vi "HFRR ADV v10.vi"() -> ()   [LabVIEW 2025] (continued)
        n1009 = property on="Analysis" class="Bool (strict)"("DisabledEnum"=w969) -> ()  [unwired: 2 in, 2 out]
        n1010 = property on="Home" class="Bool (strict)"("DisabledEnum"=w969) -> ()  [unwired: 2 in, 2 out]
        n1011 = property on="Report" class="Bool (strict)"("DisabledEnum"=w969) -> ()  [unwired: 2 in, 2 out]
        n1012 = property on="Test Setup" class="Bool (strict)"("DisabledEnum"=w969) -> ()  [unwired: 2 in, 2 out]
        n1013 = local read "Service Password enable"() -> (w967:bool)
        n1014 = case shown="True" w967 {
          tunnel: [T16."Disabled" ("Disabled") T16."Enabled" ("Disabled")] -> w966
          frame False {
          }
          frame True {
          }
        }
        n1015 = property on="About" class="Bool (strict)"("DisabledEnum"=w966) -> ()  [unwired: 2 in, 2 out]
      }
      frame "Adv Scar Report" {
        w974 = T16."Enabled" ("Disabled")
        n1016 = property on="Dashboard" class="Bool (strict)"("DisabledEnum"=T16."Disabled" ("Disabled")) -> ()  [unwired: 2 in, 2 out]
        n1017 = property on="Imaging" class="Bool (strict)"("DisabledEnum"=w974) -> ()  [unwired: 2 in, 2 out]
        n1018 = property on="Analysis" class="Bool (strict)"("DisabledEnum"=w974) -> ()  [unwired: 2 in, 2 out]
        n1019 = property on="Home" class="Bool (strict)"("DisabledEnum"=w974) -> ()  [unwired: 2 in, 2 out]
        n1020 = property on="Report" class="Bool (strict)"("DisabledEnum"=w974) -> ()  [unwired: 2 in, 2 out]
        n1021 = property on="Test Setup" class="Bool (strict)"("DisabledEnum"=w974) -> ()  [unwired: 2 in, 2 out]
        n1022 = local read "Service Password enable"() -> (w973:bool)
        n1023 = case shown="True" w973 {
          tunnel: [T16."Disabled" ("Disabled") T16."Enabled" ("Disabled")] -> w972
          frame False {
          }
          frame True {
          }
        }
        n1024 = property on="About" class="Bool (strict)"("DisabledEnum"=w972) -> ()  [unwired: 2 in, 2 out]
      }
      frame "Compare Files" {
        w980 = T16."Enabled" ("Disabled")
        n1025 = local read "Service Password enable"() -> (w979:bool)
        n1026 = property on="Dashboard" class="Bool (strict)"("DisabledEnum"=T16."Disabled" ("Disabled")) -> ()  [unwired: 2 in, 2 out]
        n1027 = property on="Imaging" class="Bool (strict)"("DisabledEnum"=w980) -> ()  [unwired: 2 in, 2 out]
        n1028 = property on="Analysis" class="Bool (strict)"("DisabledEnum"=w980) -> ()  [unwired: 2 in, 2 out]
        n1029 = property on="Home" class="Bool (strict)"("DisabledEnum"=w980) -> ()  [unwired: 2 in, 2 out]
        n1030 = property on="Report" class="Bool (strict)"("DisabledEnum"=w980) -> ()  [unwired: 2 in, 2 out]
        n1031 = property on="Test Setup" class="Bool (strict)"("DisabledEnum"=w980) -> ()  [unwired: 2 in, 2 out]
        n1032 = case shown="True" w979 {
          tunnel: [T16."Disabled" ("Disabled") T16."Enabled" ("Disabled")] -> w978
          frame False {
          }
          frame True {
          }
        }
        n1033 = property on="About" class="Bool (strict)"("DisabledEnum"=w978) -> ()  [unwired: 2 in, 2 out]
      }
      frame "Acquire" {
        n1034 = local read "Service Password enable"() -> (w984:bool)
        n1035 = property on="Test Setup" class="Bool (strict)"("DisabledEnum"=T16."Disabled" ("Disabled")) -> ()  [unwired: 2 in, 2 out]
        n1036 = local read "Auto Start Test"() -> (w986:bool)
        n1037 = local read "RUN"() -> (w988:bool)
        n1038 = case shown="True" w984 {
          tunnel: [T16."Disabled" ("Disabled") T16."Enabled" ("Disabled")] -> w985
          frame False {
          }
          frame True {
          }
        }
        n1039 = Or(x=w988, y=w986) -> (x .or. y?=w987:bool)
        n1040 = case shown="True" w987 {
          tunnel: [T16."Enabled" ("Disabled") T16."Disabled" ("Disabled")] -> w990
          frame False {
          }
          frame True {
          }
        }
        n1041 = property on="About" class="Bool (strict)"("DisabledEnum"=w985) -> ()  [unwired: 2 in, 2 out]
        n1042 = property on="Imaging" class="Bool (strict)"("DisabledEnum"=w990) -> ()  [unwired: 2 in, 2 out]
        n1043 = property on="Dashboard" class="Bool (strict)"("DisabledEnum"=w990) -> ()  [unwired: 2 in, 2 out]
        n1044 = property on="Analysis" class="Bool (strict)"("DisabledEnum"=w990) -> ()  [unwired: 2 in, 2 out]
        n1045 = property on="Home" class="Bool (strict)"("DisabledEnum"=w990) -> ()  [unwired: 2 in, 2 out]
        n1046 = property on="Report" class="Bool (strict)"("DisabledEnum"=w990) -> ()  [unwired: 2 in, 2 out]
      }
      frame "About" {
        n1047 = local read "FILE"() -> (w1003:string)
        n1048 = local read "TEST FILE NAM,E SAVED"() -> (w996:bool)
        n1049 = call <vilib>:"Trim Whitespace.vi"("string"=w1003) -> ("trimmed string"=w1002:string)  [unwired: 1 in]
        n1050 = local read "Auto Start Test"() -> (w1006:bool)
        n1051 = String Length(string=w1002) -> (length=w1001:i32)
        n1052 = Greater?(x=w1001, y=1) -> (0:w998:bool)
        n1053 = And(x=w998, y=w996) -> (x .and. y?=w997:bool)
        n1054 = local read "RUN"() -> (w1008:bool)
        n1055 = case shown="True" w997 {
          tunnel: [T16."Disabled" ("Disabled") T16."Enabled" ("Disabled")] -> w999
          frame False {
          }
          frame True {
          }
        }
        n1056 = Or(x=w1008, y=w1006) -> (x .or. y?=w1007:bool)
        n1057 = property on="About" class="Bool (strict)"("DisabledEnum"=T16."Enabled" ("Disabled")) -> ()  [unwired: 2 in, 2 out]
        n1058 = case shown="False" w1007 {
          tunnel: [T16."Enabled" ("Disabled") T16."Disabled" ("Disabled")] -> w1005
          frame False {
          }
          frame True {
          }
        }
        n1059 = property on="Dashboard" class="Bool (strict)"("DisabledEnum"=w999) -> ()  [unwired: 2 in, 2 out]
        n1060 = property on="Test Setup" class="Bool (strict)"("DisabledEnum"=T16."Disabled" ("Disabled")) -> ()  [unwired: 2 in, 2 out]
        n1061 = property on="Imaging" class="Bool (strict)"("DisabledEnum"=w1005) -> ()  [unwired: 2 in, 2 out]
        n1062 = property on="Analysis" class="Bool (strict)"("DisabledEnum"=w1005) -> ()  [unwired: 2 in, 2 out]
        n1063 = property on="Home" class="Bool (strict)"("DisabledEnum"=w1005) -> ()  [unwired: 2 in, 2 out]
        n1064 = property on="Report" class="Bool (strict)"("DisabledEnum"=w1005) -> ()  [unwired: 2 in, 2 out]
      }
    }
    n1065 = local read "Quit"() -> (w939:bool)
    "Single" <- "Single - Graph"
  }
  n1066 = disable-structure shown="Disabled" {
    disable-tunnel: [w1263 _] -> w36
    disable-tunnel: _ -> [w1262 _]
    frame Disabled {
      n1067 = while {
        tunnel: w1262 -> [_]
        tunnel: [w1264] -> w1263
        tunnel: [w1265] -> _
        i -> [w1265]
        stop <- w1264 stop-if-true
        w1281 = u16 10 items=["1.0"=10, "1.5"=15, "2.0"=20] ("stop bits (10: 1 bit)")
        n1068 = Wait (ms)(milliseconds to wait=u32 10) -> ()  [unwired: 1 out]
        n1069 = call-poly "VISA Configure Serial Port"("VISA resource name"=refnum<visa-resource-name> "ASRL1::INSTR" ("COM PORT"), "timeout (10sec)"=u32 10, "baud rate (9600)"=u32 57600, "data bits (8)"=u16 8, "stop bits (10: 1 bit)"=w1281) -> ("VISA resource name out"=w1267:refnum<visa-resource-name>, "error out"=w1276:errorcluster)  [unwired: 9 in]
        n1070 = VISA Read(VISA resource name=w1267, byte count=u32 2 ("byte count (0)")) -> (read buffer=w1275:string)  [unwired: 1 in, 3 out]
        n1071 = String Subset(string=w1275, offset (0)=0, length (rest)=2 ("length (rest)")) -> (substring=w1274:string)
        n1072 = Match Pattern(string=w1274, regular expression="<>") -> (offset past match=w1271:i32)  [unwired: 1 in, 3 out]
        n1073 = Greater Or Equal?(x=w1271, y=0) -> (x >= y?=w1266:bool)
        n1074 = case shown="True" w1266 {
          tunnel: w1267 -> [_ w1285]
          tunnel: w1276 -> [_ w1284]
          frame False {
          }
          frame True {
            n1075 = VISA Read(VISA resource name=w1285, byte count=u32 32 ("byte count (0)"), error in (no error)=w1284) -> (read buffer=w1283:string)  [unwired: 3 out]
            n1076 = String Subset(string=w1283, offset (0)=0, length (rest)=8 ("length (rest)")) -> (substring=w1287:string)
            n1077 = String Subset(string=w1283, offset (0)=8, length (rest)=8 ("length (rest)")) -> (substring=w1288:string)
            n1078 = Decimal String To Number(string=w1288) -> (number=w1295:i32)  [unwired: 2 in, 1 out]
            n1079 = Decimal String To Number(string=w1287) -> (number=w1291:i32)  [unwired: 2 in, 1 out]
            n1080 = Divide(x=w1295, y=10000) -> ()  [unwired: 1 out]
            n1081 = Divide(x=w1291, y=1000000) -> ()  [unwired: 1 out]
          }
        }
        n1082 = local read "Quit"() -> (w1264:bool)
      }
    }
    frame Enabled {
    }
  }
  n1083 = local write "Err Count"(0 ("Err Count")) -> ()
  n1084 = local write "FRICVALZ"(0.0 ("FRICVALZ")) -> ()
  n1085 = Tick Count (ms)() -> (millisecond timer value=w49:u32)
  n1086 = while {
    shift-right: [w1314] -> w53
    shift-left: _ -> [w1303]
    shift-right: [w1313] -> w52
    shift-left: errorcluster {"status"=TRUE, "code"=0, "source"="Init"} ("error IO") -> [w1305]
    shift-right: [w1311] -> _
    shift-left: w49 -> [w1312]
    tunnel: [w1298] -> w40
    tunnel: [w1310] -> _
    i -> [w1310]
    stop <- w1298 stop-if-true
    n1087 = local read "Com Port 1"() -> (w1304:refnum<visa-resource-name>)
    n1088 = local read "Port 1a"() -> (w1306:bool)
    n1089 = local read "Port 3"() -> (w1307:bool)
    n1090 = Not Equal?(x=w1304, y=w1303) -> (x != y?=w1302:bool)
    n1091 = Or(x=w1307, y=w1306) -> (x .or. y?=w1309:bool)
    n1092 = Unbundle(w1305) -> ("status"=→"Port 3":bool)  [unwired: 2 out]
    n1093 = flat-sequence {
      tunnel: [w1317] -> w1301
      tunnel: w1305 -> [w1317]
      frame #0 {
        n1094 = Wait (ms)(milliseconds to wait=u32 200) -> ()  [unwired: 1 out]
      }
    }
    n1095 = case shown="True" w1309 {
      frame False {
        w1319 = FALSE ("Visible")
        n1096 = property on="Port 1a" class="Bool (strict)"("Visible"=w1319) -> ()  [unwired: 2 in, 2 out]
        n1097 = property on="Port 3" class="Bool (strict)"("Visible"=w1319) -> ()  [unwired: 2 in, 2 out]
      }
      frame True {
        w1320 = TRUE ("Visible")
        n1098 = property on="Port 1a" class="Bool (strict)"("Visible"=w1320) -> ()  [unwired: 2 in, 2 out]
        n1099 = property on="Port 3" class="Bool (strict)"("Visible"=w1320) -> ()  [unwired: 2 in, 2 out]
      }
    }
    n1100 = Or(x=w1302, y="Re-initialize Port1") -> (x .or. y?=w1299:bool)
    n1101 = case shown="True" w1299 {
      tunnel: [w1315 errorcluster {"status"=TRUE, "code"=0, "source"="Init"} ("error out")] -> w1300
      tunnel: w1301 -> [w1315 _]
      frame False {
      }
      frame True {
      }
    }
    n1102 = case shown="No Error" w1300 {
      selector: w1300 -> [w1321 w1666]
      tunnel: [w1326 w1671] -> w1314
      tunnel: [w1325 w1663] -> w1313
      tunnel: w1303 -> [w1324 w1669]
      tunnel: w1312 -> [w1323 w1668]
      tunnel: [w1322 w1668] -> w1311
      frame No Error {
        n1103 = stacked-sequence {
          tunnel: [w1336 _ _ _ _ _] -> w1326
          tunnel: [w1335 _ _ _ _ _] -> w1325
          tunnel: w1324 -> [w1331 _ _ _ _ _]
          tunnel: w1321 -> [w1330 _ _ _ _ _]
          tunnel: w1323 -> [_ w1459 _ _ _ _]
          tunnel: [_ w1458 _ _ _ _] -> w1322
          tunnel: [_ w1430 _ _ _ _] -> _
          frame #0 {
            n1104 = property class="Instr"(reference=w1331, error in=w1330) -> (reference out=w1333:refnum<visa-resource-name>, error out=w1334:errorcluster, "Serial Settings:Number of Bytes at Serial Port"=w1327:u32)
            "Sps 3" <- w1327
            "Port 1" <- w1327
            n1105 = Greater?(x=w1327, y=u32 5) -> (0:w1329:bool)
            n1106 = case shown="True" w1329 {
              tunnel: w1333 -> [w1338 w1365]
              tunnel: w1334 -> [w1337 w1344]
              tunnel: [w1337 w1340] -> w1335
              tunnel: [w1338 w1366] -> w1336
              frame False {
              }
              frame True {
                w1339 = TRUE ("PAUSE")
                w1342 = TRUE ("PAUSE")
                # "Out as Volts"
                n1107 = call "ELAPSED TIMER VI - uno.vi"("error in"=w1344, "RESET"=w1342, "PAUSE"=w1342) -> ("error out"=w1343:errorcluster)  [unwired: 6 in, 2 out]
                n1108 = local read "Residual Uno"() -> (w1359:string)
                n1109 = while {
                  tunnel: [w1414] -> w1341
                  tunnel: [w1413] -> w1366
                  tunnel: w1343 -> [w1412]
                  tunnel: w1365 -> [w1411]
                  tunnel: [w1408] -> _
                  shift-right: [w1404] -> w1347
                  shift-left: w1359 -> [w1406]
                  i -> [w1408]
                  stop <- w1403 stop-if-true
                  w1401 = FALSE ("PAUSE")
                  n1110 = property class="Instr"(reference=w1411, error in=w1412) -> (reference out=w1416:refnum<visa-resource-name>, error out=w1415:errorcluster, "Serial Settings:Number of Bytes at Serial Port"=w1407:u32)
                  n1111 = local read "Quit"() -> (w1402:bool)
                  n1112 = call "ELAPSED TIMER VI - uno.vi"("TARGET"=5.0, "RESET"=w1401, "PAUSE"=w1401) -> ("ELAPSED INDICATION"=w1399:bool)  [unwired: 6 in, 2 out]
                  "ELAPSED INDICATION" <- w1399
                  n1113 = VISA Read(VISA resource name=w1416, byte count=w1407, error in (no error)=w1415) -> (VISA resource name out=w1413:refnum<visa-resource-name>, read buffer=w1405:string, error out=w1414:errorcluster)  [unwired: 1 out]
                  n1114 = Greater?(x=w1407, y=u32 30) -> (0:w1409:bool)
                  n1115 = Concatenate Strings(w1406, w1405) -> (w1404:string)
                  n1116 = Compound Arithmetic op=OR(w1409, w1402, w1399) -> (w1403:bool)
                }
                "UnoRead" <- w1347
                n1117 = call "ELAPSED TIMER VI - uno.vi"("error in"=w1341, "RESET"=w1339, "PAUSE"=w1339) -> ("error out"=w1340:errorcluster)  [unwired: 6 in, 2 out]
                n1118 = while {
                  shift-right: [w1385] -> w1358
                  shift-left: w1347 -> [w1391]
                  tunnel: [w1384] -> w1354 mode=indexing
                  tunnel: [w1386] -> _
                  i -> [w1386]
                  stop <- w1383 stop-if-true
                  n1119 = Match Pattern(string=w1391, regular expression="*") -> (after substring=w1389:string)  [unwired: 1 in, 3 out]
                  n1120 = local read "Quit"() -> (w1382:bool)
                  n1121 = local read "ELAPSED INDICATION"() -> (w1381:bool)
                  n1122 = Match Pattern(string=w1389, regular expression="&") -> (before substring=w1384:string, after substring=w1385:string, offset past match=w1387:i32)  [unwired: 1 in, 1 out]
                  n1123 = Less Than 0?(x=w1387) -> (x < 0?=w1388:bool)
                  n1124 = Compound Arithmetic op=OR(w1388, w1382, w1381) -> (w1383:bool)
                }
                n1125 = local write "Residual Uno"(w1358) -> ()
                n1126 = Array Size(array=w1354) -> (size(s)=w1355:i32)
                n1127 = Decrement(x=w1355) -> (x-1=w1357:i32)
                n1128 = Delete From Array(array=w1354, length=1, index=w1357) -> (array with subset deleted=w1352:string[])  [unwired: 1 out]
                n1129 = Array Size(array=w1352) -> (size(s)=w1351:i32)
                n1130 = Decrement(x=w1351) -> (x-1=w1350:i32)
                n1131 = while {
                  tunnel: [w1380] -> w1363 mode=indexing
                  tunnel: [w1379] -> w1362 mode=indexing
                  tunnel: w1352 -> [w1373] mode=indexing
                  tunnel: w1350 -> [w1372]
                  tunnel: [w1371] -> _
                  i -> [w1371]
                  stop <- w1367 stop-if-true
                  w1374 = 0 ("length (rest)")
                  w1376 = ";" ("regular expression")
                  n1132 = local read "ELAPSED INDICATION"() -> (w1370:bool)
                  n1133 = Less Or Equal?(x=w1372, y=w1371) -> (x <= y?=w1368:bool)
                  n1134 = local read "Quit"() -> (w1369:bool)
                  n1135 = Compound Arithmetic op=OR(w1368, w1369, w1370) -> (w1367:bool)
                  n1136 = Match Pattern(string=w1373, regular expression=w1376) -> (before substring=w1378:string, after substring=w1377:string)  [unwired: 1 in, 2 out]
                  n1137 = Decimal String To Number(string=w1378, default (0L)=w1374) -> (number=w1380:i32)  [unwired: 1 in, 1 out]
                  n1138 = Match Pattern(string=w1377, regular expression=w1376) -> (before substring=w1375:string)  [unwired: 1 in, 3 out]
                  n1139 = Decimal String To Number(string=w1375, default (0L)=w1374) -> (number=w1379:i32)  [unwired: 1 in, 1 out]
                }
                n1140 = case shown="0, Default" "ADC Res" {
                  tunnel: [w1394 w1396] -> w1346
                  frame 0, Default {
                    n1141 = Divide(x=65535 ("length (rest)"), y=2 ("length (rest)")) -> (x/y=w1394:dbl)
                  }
                  frame 1 {
                    n1142 = Divide(x=16777216 ("length (rest)"), y=2 ("length (rest)")) -> (x/y=w1396:dbl)
                  }
                }
                n1143 = Bundle(w1363, w1362) -> (w1353:cluster{i32[], i32[]})  [unwired: 1 in]
                n1144 = Divide(x=w1353, y=w1346) -> (x/y=w1364:cluster{dbl[], dbl[]})
                n1145 = Multiply(x=w1364, y=sgl 5.03 ("Numeric")) -> (x*y=w1361:cluster{dbl[], dbl[]})
                n1146 = Unbundle(w1361) -> (→"Ch1":dbl[], →"Ch0":dbl[])
              }
            }
            n1147 = Not(x=w1329) -> (.not. x?=→"Port 1a":bool)
          }
          frame #1 {
            n1148 = local read "zOff 2"() -> (w1451:dbl)
            n1149 = local read "Ch1"() -> (w1441:dbl[])
            n1150 = case shown="True" "Zero 2" {
              tunnel: w1441 -> [_ w1471]
              frame False {
              }
              frame True {
                n1151 = call-poly <vilib>:"Mean.vi"("X"=w1471) -> ("mean"=→"zOff 2":dbl)  [unwired: 1 out]
                n1152 = local write "Zero 2"(FALSE ("Zero")) -> ()
              }
            }
            n1153 = Subtract(x=w1441, y=w1451) -> (x-y=w1447:dbl[])
            n1154 = call-poly <vilib>:"Mean.vi"("X"=w1441) -> ("mean"=w1442:dbl)  [unwired: 1 out]
            "Slide 3" <- w1442
            n1155 = Multiply(x=w1447, y=1.0 ("PG Oth")) -> (x*y=w1433:dbl[])
            n1156 = local read "FF buffer"() -> (w1438:dbl[])
            n1157 = Divide(x=w1433, y=1) -> (x/y=w1432:dbl[])
            "Fric Val" <- w1432
            n1158 = call <vilib>:"Mean PtByPt.vi"("x"=w1442, "sample length"=10, "initialize"="Reset 2") -> ("mean"=→"Mean Pos Fil 2":dbl)  [unwired: 1 in, 1 out]
            n1159 = Array Size(array=w1438) -> (size(s)=w1440:i32)
            n1160 = call-poly <vilib>:"Mean.vi"("X"=w1432) -> ("mean"=w1446:dbl)  [unwired: 1 out]
            n1161 = Insert Into Array(array=w1438, index=w1440, new element=w1432) -> (w1435:dbl[])
            n1162 = Array Size(array=w1435) -> (size(s)=w1434:i32)
            n1163 = case shown="True" "DC corr 2" {
              tunnel: w1432 -> [w1474 w1477]
              tunnel: [w1474 w1476] -> w1439
              tunnel: w1446 -> [_ w1475]
              frame False {
              }
              frame True {
                n1164 = Subtract(x=w1477, y=w1475) -> (x-y=w1476:dbl[])
              }
            }
            n1165 = Tick Count (ms)() -> (millisecond timer value=w1458:u32)
            n1166 = Greater?(x=w1434, y=1000) -> (0:w1436:bool)
            n1167 = Subtract(x=w1458, y=w1459) -> (x-y=w1457:u32)
            n1168 = case shown="True" w1436 {
              tunnel: [w1464 w1467] -> w1423
              tunnel: w1435 -> [w1464 w1470]
              tunnel: w1434 -> [_ w1469]
              frame False {
              }
              frame True {
                n1169 = Subtract(x=w1469, y=1000) -> (x-y=w1465:i32)
                n1170 = Delete From Array(array=w1470, length=w1465, index=0) -> (array with subset deleted=w1467:dbl[])  [unwired: 1 out]
              }
            }
            n1171 = Divide(x=w1457, y=u32 1000 ("x")) -> (x/y=w1455:dbl)
            n1172 = Array Size(array=w1439) -> (size(s)=w1454:i32)
            n1173 = Divide(x=w1454, y=w1455) -> (x/y=w1450:dbl)
            "Sps 2" <- w1450
            n1174 = Reciprocal(x=w1450) -> (1/x=w1448:dbl)
            "dt" <- w1448
            n1175 = local read "FRIC. FORCE :"() -> (w1420:dbl)
            n1176 = local write "FF buffer"(w1423) -> ()
            n1177 = Negate(x=w1423) -> (-x=w1422:dbl[])
            n1178 = call "Elapsed Time5"("Time Target (s)"="check time s", "Reset"="Reset 3") -> ("Time has Elapsed"=w1425:bool)  [unwired: 10 in, 7 out]
            n1179 = Array Max & Min(array=w1422) -> (max value=w1430:dbl)  [unwired: 3 out]
            n1180 = Bundle By Name("Y"=w1439, "dt"=w1448, "t0"=timestamp(0 s since 1904-01-01)) -> (w1418:waveform(dbl))  [unwired: 1 in]
            n1181 = Multiply(x=w1420, y=21.1986) -> (x*y=w1419:dbl)
            n1182 = Greater Or Equal?(x=w1430, y="Threshold value") -> (x >= y?=w1426:bool)
            n1183 = Multiply(x=w1419, y=w1418) -> (x*y=→"FF_Wfm":waveform(dbl))
            n1184 = And(x=w1426, y=w1425) -> (x .and. y?=w1424:bool)
            n1185 = case shown="True" w1424 {
              frame False {
                n1186 = local write "Reset 3"(FALSE ("Reset 3")) -> ()
              }
              frame True {
                n1187 = local write "Reset 3"(TRUE ("Reset 3")) -> ()
                n1188 = local write "save dpt"(TRUE ("save dpt")) -> ()
              }
            }
          }
          frame #2 {
            n1189 = local read "FF buffer"() -> (w1484:dbl[])
            n1190 = Array Max & Min(array=w1484) -> (max value=w1479:dbl, min value=w1480:dbl)  [unwired: 2 out]
            n1191 = Subtract(x=w1479, y=w1480) -> (x-y=w1481:dbl)
            n1192 = Multiply(x=1.0 ("y 2"), y="Threshold") -> ()  [unwired: 1 out]
            n1193 = Greater?(x=w1481, y="Threshold") -> (0:w1478:bool)
            n1194 = case shown="True" w1478 {
              tunnel: w1484 -> [_ w1491]
              tunnel: [_ w1489] -> _
              frame False {
              }
              frame True {
                w1490 = 1.0 ("y")
                n1195 = Delete From Array(array=w1491, length=100, index=0) -> (deleted portion=w1496:dbl[])  [unwired: 1 out]
                n1196 = call-poly <vilib>:"Mean.vi"("X"=w1496) -> ("mean"=w1495:dbl)  [unwired: 1 out]
                n1197 = Subtract(x=w1491, y=w1495) -> (x-y=w1494:dbl[])
                n1198 = Multiply(x=w1490, y=w1490) -> (x*y=w1492:dbl)
                n1199 = Multiply(x=w1494, y=w1492) -> (x*y=w1493:dbl[])
                "FF cal val" <- w1493
                n1200 = Array Size(array=w1493) -> (size(s)=w1487:i32)
                n1201 = Array Max & Min(array=w1493) -> (max value=w1486:dbl, min value=w1485:dbl)  [unwired: 2 out]
                n1202 = property on="FF Calibration g" class="WFGraph (strict)"("X Scale.Range:Minimum"=0.0 ("y"), "X Scale.Range:Maximum"=w1487, "Y Scale.Range:Minimum"=w1486, "Y Scale.Range:Maximum"=w1485) -> ()  [unwired: 2 in, 2 out]
                n1203 = local read "FRIC. FORCE :"() -> (w1489:dbl)
              }
            }
          }
          frame #3 {
            # "5"
            n1204 = local read "DISPLACEMENT :"() -> (w1587:dbl)
            n1205 = Multiply(x=w1587, y=1.0) -> (x*y=w1505:dbl)
            n1206 = local read "zOff 3"() -> (w1590:dbl)
            n1207 = local read "Ch0"() -> (w1518:dbl[])
            n1208 = case shown="True" "Zero 3" {
              tunnel: w1518 -> [_ w1605]
              frame False {
              }
              frame True {
                n1209 = call-poly <vilib>:"Mean.vi"("X"=w1605) -> ("mean"=→"zOff 3":dbl)  [unwired: 1 out]
                n1210 = local write "Zero 3"(FALSE ("Zero")) -> ()
              }
            }
            n1211 = Add(x=w1518, y="Offset") -> (x+y=w1517:dbl[])
            n1212 = Multiply(x=w1505, y="DISPLACEMENT : 2") -> (x*y=w1572:dbl)
            n1213 = Subtract(x=w1518, y=w1590) -> (x-y=w1575:dbl[])
            n1214 = Multiply(x=w1575, y=w1572) -> (x*y=w1574:dbl[])
            n1215 = Multiply(x=w1575, y=w1505) -> (x*y=w1586:dbl[])
            "ABS DP" <- w1586
            n1216 = local read "Standard Slip Gauge (mm)"() -> (w1573:dbl)
            n1217 = call-poly <vilib>:"Mean.vi"("X"=w1574) -> ("mean"=w1504:dbl)  [unwired: 1 out]
            "Disp (mm)" <- w1504
            "software msrnt" <- w1504
            n1218 = Multiply(x=w1517, y="Gain") -> (x*y=w1512:dbl[])
            "Voltage LVDT Acq" <- w1512
            "gLVDTraw" <- w1512
            n1219 = call-poly <vilib>:"Mean.vi"("X"=w1586) -> ("mean"=w1577:dbl)  [unwired: 1 out]
            n1220 = case shown="True" "DC correction" {
              tunnel: w1586 -> [w1608 w1611]
              tunnel: [w1608 w1610] -> w1524
              tunnel: w1577 -> [_ w1609]
              frame False {
              }
              frame True {
                n1221 = Subtract(x=w1611, y=w1609) -> (x-y=w1610:dbl[])
              }
            }
            n1222 = Divide(x=w1504, y=w1573) -> (x/y=w1571:dbl)
            n1223 = call-poly <vilib>:"Mean.vi"("X"=w1512) -> ("mean"=w1511:dbl)  [unwired: 1 out]
            n1224 = Array Max & Min(array=w1512) -> (max value=w1516:dbl, min value=w1515:dbl)  [unwired: 2 out]
            n1225 = Multiply(x=w1571, y=w1572) -> (x*y=→"DISPLACEMENT : 3":dbl)
            n1226 = Subtract(x=w1516, y=w1515) -> (x-y=→"Pk-Pk":dbl)
            n1227 = local read "dt"() -> (w1589:dbl)
            n1228 = Threshold 1D Array(2:0.0 ("threshold y"), 3:w1524) -> (0:w1541:dbl)  [unwired: 1 in]
            n1229 = Bundle By Name("Y"=w1524, "dt"=w1589, "t0"=timestamp(0 s since 1904-01-01)) -> (w1579:waveform(dbl))  [unwired: 1 in]
            n1230 = local read "FF_Wfm"() -> (w1578:waveform(dbl))
            n1231 = Equal To 0?(x=w1541) -> (x = 0?=w1542:bool)
            n1232 = case shown="True" w1542 {
              tunnel: w1524 -> [_ w1599]
              tunnel: [w1595 w1596] -> w1537
              tunnel: w1541 -> [w1595 _]
              frame False {
              }
              frame True {
                n1233 = Threshold 1D Array(1:20 ("start index (0)"), 2:0.0 ("threshold y"), 3:w1599) -> (0:w1596:dbl)
              }
            }
            n1234 = Build Array(w1579, w1578) -> (w1560:waveform(dbl)[])
            "Waveform Graph 2" <- w1560
            n1235 = call-poly <vilib>:"Extract Single Tone Information.vi"("time signal in"=w1579) -> ("detected amplitude"=w1513:dbl, "detected frequency"=→"RawFreq":dbl)  [unwired: 5 in, 4 out]
            n1236 = Multiply(x=w1513, y=2.0) -> (x*y=w1500:dbl)
            n1237 = Subtract(x=w1511, y="LvdtOff") -> (x-y=w1510:dbl)
            n1238 = local read "StrokeL"() -> (w1501:dbl)
            n1239 = Not A Number/Path/Refnum?(number/path/refnum=w1500) -> (NaN/Path/Refnum?=w1502:bool)
            n1240 = Subtract(x=w1510, y=w1513) -> (x-y=w1522:dbl)
            n1241 = Add(x=w1513, y=w1510) -> (x+y=w1521:dbl)
            n1242 = Index Array(array=w1560) -> (element #1=w1561:waveform(dbl), element #2=w1563:waveform(dbl))  [unwired: 2 in]
            n1243 = Select(t=w1501, s=w1502, f=w1500) -> (s? t:f=w1499:dbl)
            "Stroke" <- w1499
            "Mean(RAW) Stroke" <- w1499
            "StrokeL" <- w1499
            n1244 = Bundle(w1510, w1522, w1521) -> (→"Slide 8":cluster{dbl, dbl, dbl})  [unwired: 1 in]
            n1245 = Unbundle By Name(w1561) -> ("Y"=w1534:dbl[])
            n1246 = Split 1D Array(array=w1524, index=w1537) -> (second subarray=w1538:dbl[])  [unwired: 1 out]
            n1247 = In Range and Coerce(upper limit=1.5, x=w1499, lower limit=0.5) -> (In Range?=w1583:bool)  [unwired: 1 out]
            n1248 = Split 1D Array(array=w1534, index="Window") -> (second subarray=w1552:dbl[])  [unwired: 1 out]
            n1249 = Unbundle By Name(w1563) -> ("Y"=w1535:dbl[])
            n1250 = Threshold 1D Array(1:180 ("start index (0)"), 2:0.0 ("threshold y"), 3:w1538) -> (0:w1536:dbl)
            n1251 = local read "Test \nStatus"() -> (w1580:bool)
            n1252 = Split 1D Array(array=w1535, index=w1537) -> (second subarray=w1532:dbl[])  [unwired: 1 out]
            n1253 = Not(x=w1583) -> (.not. x?=w1582:bool)
            n1254 = call-poly <vilib>:"RMS.vi"("X"=w1552) -> ("rms value"=w1508:dbl)  [unwired: 1 out]
            "Current (A)" <- w1508
            n1255 = Array Max & Min(array=w1552) -> (max value=w1566:dbl, min value=w1567:dbl)  [unwired: 2 out]
            n1256 = Array Max & Min(array=w1535) -> (max value=w1564:dbl, min value=w1565:dbl)  [unwired: 2 out]
            n1257 = Subtract(x=w1566, y=w1567) -> (x-y=w1568:dbl)
            n1258 = Subtract(x=w1564, y=w1565) -> (x-y=w1569:dbl)
            n1259 = And(x=w1582, y=w1580) -> (x .and. y?=w1581:bool)
            n1260 = Split 1D Array(array=w1538, index=w1536) -> (first subarray=w1531:dbl[])  [unwired: 1 out]
            n1261 = Split 1D Array(array=w1532, index=w1536) -> (first subarray=w1529:dbl[])  [unwired: 1 out]
            n1262 = case shown="True" w1581 {
              tunnel: [i32[] [] w1601] -> _
              frame False {
              }
              frame True {
                n1263 = local read "UnoRead"() -> (w1603:string)
                n1264 = local read "Array"() -> (w1604:string[])
                n1265 = Build Array (concatenate)(w1604, w1603) -> (w1602:string[])
                "Array" <- w1602
                n1266 = String Length(string=w1602) -> (length=w1601:i32[])
              }
            }
            n1267 = local read "G_val"() -> (w1554:dbl)
            n1268 = Divide(x=w1569, y=w1568) -> (x/y=w1557:dbl)
            n1269 = call-poly <vilib>:"RMS.vi"("X"=w1529) -> ("rms value"=w1553:dbl)  [unwired: 1 out]
            n1270 = call-poly <vilib>:"Hanning Window.vi"("X"=w1531) -> ("Windowed X"=w1530:dbl[])  [unwired: 1 out]
            n1271 = call-poly <vilib>:"Hanning Window.vi"("X"=w1529) -> ("Windowed X"=w1528:dbl[])  [unwired: 1 out]
            n1272 = local read "Constant (G)"() -> (w1546:dbl)
            n1273 = Divide(x=w1553, y=w1508) -> (x/y=w1547:dbl)
            n1274 = Build Array(w1530, w1528) -> (→"Waveform Graph 4":dbl[][])
            n1275 = Multiply(x=w1557, y=0.2) -> (x*y=w1559:dbl)
            n1276 = Multiply(x=0.8 ("y"), y=w1554) -> (x*y=w1558:dbl)
            n1277 = Add(x=w1559, y=w1558) -> (x+y=w1526:dbl)
            n1278 = Multiply(x=w1547, y=0.2) -> (x*y=w1548:dbl)
            n1279 = Multiply(x=0.8 ("y"), y=w1546) -> (x*y=w1549:dbl)
            n1280 = Add(x=w1548, y=w1549) -> (x+y=w1545:dbl)
            "Constant (G)" <- w1545
            n1281 = Not A Number/Path/Refnum?(number/path/refnum=w1526) -> (NaN/Path/Refnum?=w1525:bool)
            n1282 = Select(t=0.0, s=w1525, f=w1526) -> (s? t:f=w1506:dbl)
            "G_val" <- w1506
            n1283 = Multiply(x=w1508, y=w1506) -> (x*y=→"Friction Force (N)":dbl)
            n1284 = Bundle(w1545, "t"=w1506) -> (→"pk-pk":cluster{dbl, "t":dbl})  [unwired: 1 in]
          }
          frame #4 {
            # "C:\\WinDucom\\data\\"
            # "?C:\\LAB-IQ-NXT\\data"
            n1285 = case shown="True" "save dpt" {
              frame False {
              }
              frame True {
                n1286 = local write "save dpt"(FALSE ("Hold 3")) -> ()
                n1287 = local read "file count"() -> (w1615:i32)
                n1288 = Number To Decimal String(number=w1615) -> (decimal integer string=w1621:string)  [unwired: 1 in]
                n1289 = Add(x=1, y=w1615) -> (x+y=w1616:i32)
                n1290 = local write "file count"(w1616) -> ()
                n1291 = local read "FILE 2"() -> (w1620:string)
                n1292 = Concatenate Strings(w1620, w1621) -> (w1613:string)
                n1293 = Concatenate Strings("C:\\LAB-IQ\\data" ("Substring"), w1613) -> (w1628:string)
                n1294 = local read "FF buffer"() -> (w1623:dbl[])
                n1295 = local read "ABS DP"() -> (w1622:dbl[])
                n1296 = Concatenate Strings(w1628, ".dpf" ("Substring")) -> (w1626:string)
                n1297 = Build Array(w1623, w1622) -> (w1618:dbl[][])
                n1298 = Concatenate Strings("FF ( V ); DP( mincron ) " ("character string"), "\r") -> (w1632:string)
                n1299 = String To Path(string=w1626) -> (path=w1624:path)
                n1300 = Transpose 2D Array(2D array=w1618) -> (transposed array=w1617:dbl[][])
                n1301 = call <vilib>:"Write Characters To File.vi"("append to file? (new file:F)"=FALSE, "character string"=w1632, "file path (dialog if empty)"=w1624) -> ("new file path (Not A Path if cancelled)"=w1629:path)  [unwired: 2 in]
                n1302 = Array To Spreadsheet String(delimiter (Tab)=";", array=w1617, 3:"" ("format string")) -> (spreadsheet string=w1619:string)
                "String 9" <- w1619
                n1303 = call <vilib>:"Write Characters To File.vi"("append to file? (new file:F)"=TRUE, "character string"=w1619, "file path (dialog if empty)"=w1629) -> ()  [unwired: 2 in, 1 out]
              }
            }
          }
          frame #5 {
            n1304 = case shown="True" "Hold 4" {
              frame False {
              }
              frame True {
                n1305 = File Dialog(6:"*.dpf" ("pattern"), 11:path "C:/LAB-IQ" ("start path")) -> (0:w1639:errorcluster, 3:w1654:path)  [unwired: 5 in, 2 out]
                n1306 = Unbundle(w1639) -> ()  [unwired: 3 out]
                n1307 = call <vilib>:"Read Characters From File.vi"("file path (dialog if empty)"=w1654) -> ("character string"=w1644:string)  [unwired: 5 in, 3 out]
                n1308 = Spreadsheet String To Array(delimiter (Tab)=";", format string="%S", spreadsheet string=w1644, array type (2D Dbl)=string[][] []) -> (array=w1648:string[][])
                n1309 = for {
                  tunnel: w1648 -> [w1658] mode=indexing
                  tunnel: [w1657] -> w1649 mode=indexing
                  n1310 = for {
                    tunnel: w1658 -> [w1660] mode=indexing
                    tunnel: [w1659] -> w1657 mode=indexing
                    n1311 = call <vilib>:"Trim Whitespace.vi"("string"=w1660) -> ("trimmed string"=w1659:string)  [unwired: 1 in]
                  }
                }
                n1312 = Fract/Exp String To Number(string=w1649) -> (number=w1651:dbl[][])  [unwired: 3 in, 1 out]
                n1313 = Array Subset(array=w1651, index (row)=1 ("index (col)")) -> (w1653:dbl[][])  [unwired: 3 in]
                n1314 = Index Array(array=w1653, index (col) #1=0 ("disabled index (col)"), index (col) #2=1 ("disabled index (col)")) -> (element #1=w1642:dbl[], element #2=w1641:dbl[])  [unwired: 2 in]
                n1315 = Build Array(w1642, w1641) -> (→"Waveform Graph":dbl[][])
              }
            }
          }
        }
      }
      frame Error {
        w1677 = u16 0 items=["None", "XON/XOFF", "RTS/CTS", "XON/XOFF & RTS/CTS", "DTR/DSR", "XON/XOFF & DTR/DSR"] ("flow control (0:none)  2")
        w1675 = u16 10 items=["1.0"=10, "1.5"=15, "2.0"=20] ("stop bits 2")
        w1673 = u16 0 items=["None", "Odd", "Even", "Mark", "Space"] ("parity 2")
        w1674 = u32 10000  # timeout (10sec)
        n1316 = VISA Close(VISA resource name=w1669, error in (no error)=w1666) -> (error out=w1670:errorcluster)
        n1317 = local write "Sps 3"(0.0 ("Sps 4")) -> ()
        n1318 = local write "Port 1a"(FALSE ("Port 1a")) -> ()
        n1319 = call <vilib>:"Clear Errors.vi"("error in (no error)"=w1670) -> ("error out"=w1667:errorcluster)  [unwired: 5 in, 1 out]
        n1320 = local read "Com Port 1"() -> (w1662:refnum<visa-resource-name>)
        n1321 = call-poly "VISA Configure Serial Port"("VISA resource name"=w1662, "timeout (10sec)"=w1674, "baud rate (9600)"=u32 250000 ("baud rate  2"), "data bits (8)"=u16 8 ("data bits  2"), "parity (0:none)"=w1673, "error in (no error)"=w1667, "stop bits (10: 1 bit)"=w1675, "flow control (0:none)"=w1677) -> ("VISA resource name out"=w1678:refnum<visa-resource-name>, "error out"=w1679:errorcluster)  [unwired: 6 in]
        n1322 = flat-sequence {
          tunnel: w1678 -> [w1681]
          tunnel: w1679 -> [w1680]
          tunnel: [w1681] -> w1671
          tunnel: [w1680] -> w1663
          frame #0 {
            n1323 = Wait (ms)(milliseconds to wait=u32 50) -> ()  [unwired: 1 out]
          }
        }
        "Residual Uno" <- ""
        "Port 1 Error" <- w1663
      }
    }
    n1324 = local read "Quit"() -> (w1298:bool)
    "Error Uno" <- w1305
  }
  n1325 = while {
    shift-right: [w1698] -> w34
    shift-left: _ -> [w1689]
    shift-right: [w1697] -> w33
    shift-left: errorcluster {"status"=FALSE, "code"=0, "source"="Init"} ("error out") -> [w1691]
    tunnel: [w1684] -> w39
    tunnel: [w1696] -> _
    i -> [w1696]
    stop <- w1684 stop-if-true
    n1326 = local read "Com Port 2"() -> (w1690:refnum<visa-resource-name>)
    n1327 = local read "Port 2a"() -> (w1692:bool)
    n1328 = local read "Port 4"() -> (w1693:bool)
    n1329 = Not Equal?(x=w1690, y=w1689) -> (x != y?=w1688:bool)
    n1330 = Or(x=w1693, y=w1692) -> (x .or. y?=w1695:bool)
    n1331 = Unbundle(w1691) -> ("status"=→"Port 4":bool)  [unwired: 2 out]
    n1332 = flat-sequence {
      tunnel: w1691 -> [w1702]
      tunnel: [w1702] -> w1687
      frame #0 {
        n1333 = Wait (ms)(milliseconds to wait=u32 50) -> ()  [unwired: 1 out]
      }
    }
    n1334 = case shown="True" w1695 {
      frame False {
        w1703 = FALSE ("Visible")
        n1335 = property on="Port 2a" class="Bool (strict)"("Visible"=w1703) -> ()  [unwired: 2 in, 2 out]
        n1336 = property on="Port 4" class="Bool (strict)"("Visible"=w1703) -> ()  [unwired: 2 in, 2 out]
      }
      frame True {
        w1704 = TRUE ("Visible")
        n1337 = property on="Port 2a" class="Bool (strict)"("Visible"=w1704) -> ()  [unwired: 2 in, 2 out]
        n1338 = property on="Port 4" class="Bool (strict)"("Visible"=w1704) -> ()  [unwired: 2 in, 2 out]
      }
    }
    n1339 = Or(x=w1688, y="Re-initialize Port2") -> (x .or. y?=w1685:bool)
    n1340 = case shown="True" w1685 {
      tunnel: [w1699 errorcluster {"status"=TRUE, "code"=0, "source"="Init"} ("error out")] -> w1686
      tunnel: w1687 -> [w1699 _]
      frame False {
      }
      frame True {
      }
    }
    n1341 = case shown="No Error" w1686 {
      selector: w1686 -> [w1705 w1865]
      tunnel: [w1707 w1870] -> w1698
      tunnel: [w1706 w1863] -> w1697
      tunnel: w1689 -> [w1709 w1868]
      tunnel: [w1708 _] -> _
      frame No Error {
        n1342 = stacked-sequence {
          tunnel: w1709 -> [w1733 _]
          tunnel: w1705 -> [w1732 _]
          tunnel: [w1719 _] -> w1708
          tunnel: [w1718 _] -> w1707
          tunnel: [w1717 _] -> w1706
          frame #0 {
            n1343 = property class="Instr"(reference=w1733, error in=w1732) -> (reference out=w1716:refnum<visa-resource-name>, error out=w1731:errorcluster, "Serial Settings:Number of Bytes at Serial Port"=w1712:u32)
            "Port 2" <- w1712
            n1344 = Greater?(x=w1712, y=u32 23) -> (0:w1714:bool)
            n1345 = Not(x=w1714) -> ()  [unwired: 1 out]
            n1346 = case shown="True" w1714 {
              tunnel: w1716 -> [w1748 w1773]
              tunnel: w1731 -> [w1747 w1774]
              tunnel: [w1747 w1776] -> w1727
              tunnel: [w1748 w1775] -> w1728
              frame False {
              }
              frame True {
                # "Out as Volts"
                n1347 = local read "Residual Due"() -> (w1772:string)
                n1348 = while {
                  tunnel: [w1822] -> w1776
                  tunnel: [w1821] -> w1775
                  tunnel: w1774 -> [w1820]
                  tunnel: w1773 -> [w1819]
                  tunnel: [w1816] -> _
                  shift-right: [w1814] -> w1771
                  shift-left: w1772 -> [w1813]
                  i -> [w1816]
                  stop <- w1811 stop-if-true
                  n1349 = property class="Instr"(reference=w1819, error in=w1820) -> (reference out=w1824:refnum<visa-resource-name>, error out=w1823:errorcluster, "Serial Settings:Number of Bytes at Serial Port"=w1815:u32)
                  n1350 = local read "Quit"() -> (w1810:bool)
                  n1351 = VISA Read(VISA resource name=w1824, byte count=w1815, error in (no error)=w1823) -> (VISA resource name out=w1821:refnum<visa-resource-name>, read buffer=w1812:string, error out=w1822:errorcluster)  [unwired: 1 out]
                  n1352 = Greater?(x=w1815, y=u32 8) -> (0:w1817:bool)
                  n1353 = Compound Arithmetic op=OR(w1817, w1810) -> (w1811:bool)
                  n1354 = Concatenate Strings(w1813, w1812) -> (w1814:string)
                }
                n1355 = while {
                  shift-right: [w1803] -> w1755
                  shift-left: w1771 -> [w1808]
                  tunnel: [w1802] -> w1767 mode=indexing
                  tunnel: [w1801] -> _
                  i -> [w1801]
                  stop <- w1800 stop-if-true
                  n1356 = Match Pattern(string=w1808, regular expression="*") -> (after substring=w1806:string)  [unwired: 1 in, 3 out]
                  n1357 = local read "Quit"() -> (w1799:bool)
                  n1358 = Match Pattern(string=w1806, regular expression="&") -> (before substring=w1802:string, after substring=w1803:string, offset past match=w1804:i32)  [unwired: 1 in, 1 out]
                  n1359 = Less Than 0?(x=w1804) -> (x < 0?=w1805:bool)
                  n1360 = Compound Arithmetic op=OR(w1805, w1799) -> (w1800:bool)
                }
                n1361 = Array Size(array=w1767) -> (size(s)=w1770:i32)
                n1362 = local write "Residual Due"(w1755) -> ()
                n1363 = Decrement(x=w1770) -> (x-1=w1768:i32)
                n1364 = Delete From Array(array=w1767, length=1, index=w1768) -> (array with subset deleted=w1766:string[])  [unwired: 1 out]
                n1365 = Array Size(array=w1766) -> (size(s)=w1754:i32)
                n1366 = Decrement(x=w1754) -> (x-1=w1753:i32)
                n1367 = while {
                  tunnel: w1766 -> [w1787] mode=indexing
                  tunnel: w1753 -> [w1786]
                  tunnel: [w1784] -> w1761 mode=indexing
                  tunnel: [w1783] -> w1760 mode=indexing
                  tunnel: [w1782] -> w1759 mode=indexing
                  tunnel: [w1781] -> w1758 mode=indexing
                  tunnel: [w1780] -> w1756 mode=indexing
                  tunnel: [w1779] -> _
                  i -> [w1779]
                  stop <- w1778 stop-if-true
                  w1796 = u32 0 ("length (rest)")
                  w1795 = ";" ("regular expression")
                  n1368 = Less Or Equal?(x=w1786, y=w1779) -> (x <= y?=w1785:bool)
                  n1369 = Match Pattern(string=w1787, regular expression=w1795) -> (before substring=w1788:string, after substring=w1789:string)  [unwired: 1 in, 2 out]
                  n1370 = Match Pattern(string=w1789, regular expression=w1795) -> (before substring=w1792:string, after substring=w1790:string)  [unwired: 1 in, 2 out]
                  n1371 = local read "Quit"() -> (w1777:bool)
                  n1372 = Decimal String To Number(string=w1788, default (0L)=w1796) -> (number=w1784:u32)  [unwired: 1 in, 1 out]
                  n1373 = Decimal String To Number(string=w1792, default (0L)=w1796) -> (number=w1783:u32)  [unwired: 1 in, 1 out]
                  n1374 = Match Pattern(string=w1790, regular expression=w1795) -> (before substring=w1793:string, after substring=w1791:string)  [unwired: 1 in, 2 out]
                  n1375 = Decimal String To Number(string=w1793, default (0L)=w1796) -> (number=w1782:u32)  [unwired: 1 in, 1 out]
                  n1376 = Match Pattern(string=w1791, regular expression=w1795) -> (before substring=w1794:string, after substring=w1798:string)  [unwired: 1 in, 2 out]
                  n1377 = Compound Arithmetic op=OR(w1785, w1777) -> (w1778:bool)
                  n1378 = Decimal String To Number(string=w1794, default (0L)=w1796) -> (number=w1781:u32)  [unwired: 1 in, 1 out]
                  n1379 = Decimal String To Number(string=w1798, default (0L)=u8 0 ("length (rest)")) -> (number=w1780:u8)  [unwired: 1 in, 1 out]
                }
                "Din" <- w1756
                n1380 = Bundle(w1761, w1760, w1759, w1758) -> (w1763:cluster{u32[], u32[], u32[], u32[]})  [unwired: 1 in]
                n1381 = Divide(x=w1763, y=4095 ("length (rest)")) -> (x/y=w1765:cluster{dbl[], dbl[], dbl[], dbl[]})
                n1382 = Multiply(x=w1765, y=sgl 3.32 ("Numeric")) -> (x*y=w1757:cluster{dbl[], dbl[], dbl[], dbl[]})
                n1383 = Unbundle(w1757) -> (→"ECR":dbl[], →"Rtemp":dbl[], →"Air temp":dbl[], →"Ch3 2":dbl[])
              }
            }
            n1384 = call "Elapsed Time10"("Time Target (s)"=2.0, "Reset"=w1714, "Auto Reset"=FALSE) -> ("Time has Elapsed"=→"Port 2a":bool)  [unwired: 9 in, 7 out]
            n1385 = local read "Due Com"() -> (w1720:string[])
            n1386 = Array Size(array=w1720) -> (size(s)=w1719:i32)
            n1387 = Delete From Array(array=w1720, length=1, index=0) -> (deleted portion=w1723:string[], array with subset deleted=w1724:string[])
            n1388 = local write "Due Com"(w1724) -> ()
            n1389 = Index Array(array=w1723, index=0) -> (element=w1721:string)
            n1390 = Not Equal?(x=w1721, y="") -> (x != y?=w1729:bool)
            n1391 = case shown="True" w1729 {
              tunnel: w1728 -> [w1735 w1740]
              tunnel: [w1735 w1744] -> w1718
              tunnel: w1727 -> [w1734 w1739]
              tunnel: [w1734 w1742] -> w1717
              tunnel: w1721 -> [_ w1738]
              tunnel: [_ w1741] -> _
              frame False {
                # "DATA  WRITE LOOP"
              }
              frame True {
                n1392 = Concatenate Strings(w1738, "\r\n") -> (w1737:string)
                n1393 = VISA Write(VISA resource name=w1740, write buffer=w1737, error in (no error)=w1739) -> (VISA resource name out=w1744:refnum<visa-resource-name>, return count=w1741:u32, error out=w1743:errorcluster)
                n1394 = flat-sequence {
                  tunnel: w1743 -> [w1745]
                  tunnel: [w1745] -> w1742
                  frame #0 {
                    n1395 = Wait (ms)(milliseconds to wait=u32 5) -> ()  [unwired: 1 out]
                  }
                }
              }
            }
          }
          frame #1 {
            w1833 = 10 ("y")
            w1838 = 10 ("y")
            n1396 = local read "Rtemp"() -> (w1826:dbl[])
            n1397 = local read "ecr buf"() -> (w1827:dbl[])
            n1398 = for {
              tunnel: w1826 -> [w1850] mode=indexing
              shift-right: [w1851] -> w1834
              shift-left: dbl[] [] ("temp buf 2") -> [w1852]
              n1399 = Build Array (concatenate)(w1852, w1850) -> (w1853:dbl[])
              n1400 = Equal To 0?(x=w1850) -> (x = 0?=w1854:bool)
              n1401 = Select(t=w1852, s=w1854, f=w1853) -> (s? t:f=w1851:dbl[])
            }
            n1402 = local read "ECR"() -> (w1825:dbl[])
            n1403 = Insert Into Array(array=w1825, index=0, new element=w1827) -> (w1831:dbl[])
            n1404 = local read "temp buf"() -> (w1835:dbl[])
            n1405 = Array Size(array=w1831) -> (size(s)=w1832:i32)
            n1406 = Greater?(x=w1832, y=w1833) -> (0:w1830:bool)
            n1407 = case shown="True" w1830 {
              tunnel: w1831 -> [w1843 w1849]
              tunnel: w1832 -> [_ w1847]
              tunnel: w1833 -> [_ w1846]
              tunnel: [w1843 w1844] -> w1828
              frame False {
              }
              frame True {
                n1408 = Subtract(x=w1847, y=w1846) -> (x-y=w1845:i32)
                n1409 = Delete From Array(array=w1849, length=w1845, index=0) -> (array with subset deleted=w1844:dbl[])  [unwired: 1 out]
              }
            }
            "ecr buf" <- w1828
            n1410 = Insert Into Array(array=w1834, index=0, new element=w1835) -> (w1840:dbl[])
            n1411 = Array Size(array=w1840) -> (size(s)=w1839:i32)
            n1412 = Greater?(x=w1839, y=w1838) -> (0:w1841:bool)
            n1413 = case shown="True" w1841 {
              tunnel: w1840 -> [w1855 w1861]
              tunnel: w1839 -> [_ w1859]
              tunnel: w1838 -> [_ w1858]
              tunnel: [w1855 w1856] -> w1837
              frame False {
              }
              frame True {
                n1414 = Subtract(x=w1859, y=w1858) -> (x-y=w1857:i32)
                n1415 = Delete From Array(array=w1861, length=w1857, index=0) -> (array with subset deleted=w1856:dbl[])  [unwired: 1 out]
              }
            }
            "temp buf" <- w1837
          }
        }
      }
      frame Error {
        w1876 = u16 0 items=["None", "XON/XOFF", "RTS/CTS", "XON/XOFF & RTS/CTS", "DTR/DSR", "XON/XOFF & DTR/DSR"] ("flow control (0:none)  2")
        w1874 = u16 10 items=["1.0"=10, "1.5"=15, "2.0"=20] ("stop bits 2")
        w1872 = u16 0 items=["None", "Odd", "Even", "Mark", "Space"] ("parity 2")
        w1873 = u32 10000  # timeout (10sec)
        n1416 = VISA Clear(VISA resource name=w1868, error in (no error)=w1865) -> (VISA resource name out=w1867:refnum<visa-resource-name>, error out=w1866:errorcluster)
        n1417 = VISA Close(VISA resource name=w1867, error in (no error)=w1866) -> (error out=w1869:errorcluster)
        n1418 = call <vilib>:"Clear Errors.vi"("error in (no error)"=w1869) -> ()  [unwired: 5 in, 2 out]
        n1419 = local read "Com Port 2"() -> (w1862:refnum<visa-resource-name>)
        "visa due" <- w1862
        n1420 = call-poly "VISA Configure Serial Port"("VISA resource name"=w1862, "timeout (10sec)"=w1873, "baud rate (9600)"=u32 250000 ("baud rate  2"), "data bits (8)"=u16 8 ("data bits  2"), "parity (0:none)"=w1872, "stop bits (10: 1 bit)"=w1874, "flow control (0:none)"=w1876) -> ("VISA resource name out"=w1877:refnum<visa-resource-name>, "error out"=w1878:errorcluster)  [unwired: 7 in]
        n1421 = flat-sequence {
          tunnel: w1877 -> [w1880]
          tunnel: w1878 -> [w1879]
          tunnel: [w1880] -> w1870
          tunnel: [w1879] -> w1863
          frame #0 {
            n1422 = Wait (ms)(milliseconds to wait=u32 50) -> ()  [unwired: 1 out]
          }
        }
        "Residual Due" <- ""
        "Port 2 Error" <- w1863
      }
    }
    n1423 = local read "Quit"() -> (w1684:bool)
    "Error Due" <- w1691
  }
  n1424 = property on="RUN" class="Bool (strict)"("Visible"=TRUE) -> ()  [unwired: 2 in, 2 out]
  n1425 = while {
    tunnel: [w1898] -> _
    tunnel: [w1882] -> w55
    i -> [w1898]
    stop <- w1882 stop-if-true
    n1426 = local read "conststatus"() -> (w1886:dbl)
    n1427 = local read "Main Tab"() -> (w1884:T2)
    n1428 = local read "EDIT"() -> (w1904:bool)
    n1429 = local read "Rate"() -> (w1903:dbl)
    n1430 = case shown="True" w1904 {
      tunnel: [FALSE TRUE] -> w1890
      frame False {
      }
      frame True {
      }
    }
    n1431 = property on="Time slide" class="Slide (strict)"("Scale.Range:Maximum"=2500.0) -> ()  [unwired: 2 in, 2 out]
    n1432 = Equal?(x=w1884, y=T23."About" ("Main Tab")) -> (x = y?=w1896:bool)
    n1433 = Equal?(x=w1886, y=0.0) -> (x = y?=w1887:bool)
    n1434 = Divide(x=1.0, y=w1903) -> (x/y=w1899:dbl)
    "Time 2" <- w1899
    n1435 = case shown="True" w1887 {
      frame False {
      }
      frame True {
        # "C:\\WinDucom\\calibrate WO 2391.dcf"
        n1436 = local write "Lan flag"(22) -> ()
        n1437 = local write "conststatus"(10.0 ("rpm value : 2")) -> ()
        n1438 = String To Path(string="C:\\LAB-IQ\\calibrate WO 2465.dcf") -> (path=w1910:path)
        n1439 = Open/Create/Replace File "Open File"(file path (use dialog)=w1910) -> (refnum out=w1908:refnum<file>)  [unwired: 5 in, 2 out]
        n1440 = for {
          N: 23 -> [_]
          tunnel: w1908 -> [w1919]
          i -> [w1913]
          (unwired) TRUE ("line mode (F)")
          n1441 = Read from Text File "Read File"(file (use dialog)=w1919) -> (text=w1918:string)  [unwired: 3 in, 3 out]
          n1442 = Match Pattern(string=w1918, regular expression="]") -> (after substring=w1916:string)  [unwired: 1 in, 3 out]
          n1443 = String Subset(string=w1918, offset (0)=5, length (rest)=10 ("length (rest)")) -> (substring=w1911:string)
          n1444 = Fract/Exp String To Number(string=w1911) -> (number=w1912:dbl)  [unwired: 3 in, 1 out]
          n1445 = Match Pattern(string=w1916, regular expression="-") -> (before substring=w1914:string)  [unwired: 1 in, 3 out]
          n1446 = case shown="8" w1913 {
            tunnel: w1912 -> [w1922 w1923 w1924 w1925 _ _ _ w1930 w1931 w1932 w1935 w1936 w1937 w1938 w1939 w1940 w1941 w1944 w1945 _ _ w1948 _ _]
            tunnel: w1914 -> [_ _ _ _ w1926 w1927 w1928 _ _ _ _ _ _ _ _ _ _ _ _ w1946 w1947 _ w1949 _]
            frame 0 {
              n1447 = local write "FRIC. FORCE :"(w1922) -> ()
            }
            frame 1 {
              n1448 = local write "TEMPERATURE :"(w1923) -> ()
            }
            frame 2 {
              n1449 = local write "HUMIDITY:"(w1924) -> ()
            }
            frame 3 {
              n1450 = local write "AIR TEMPERATURE :"(w1925) -> ()
            }
            frame 4 {
              n1451 = local write "Com Port 1"(w1926) -> ()
            }
            frame 5 {
              n1452 = local write "Com Port 2"(w1927) -> ()
              n1453 = local write "visa due"(w1927) -> ()
            }
            frame 6 {
              n1454 = String To Path(string=w1928) -> (path=w1929:path)
              n1455 = local write "File Path"(w1929) -> ()
              "String" <- w1928
            }
            frame 7 {
              n1456 = local write "DISPLACEMENT :"(w1930) -> ()
            }
            frame 8 {
              n1457 = local write "STROKE GAIN :"(w1931) -> ()
            }
            frame 9 {
              n1458 = local read "Stroke PID Gains"() -> (w1934:T9)
              n1459 = Bundle By Name(cluster=w1934, "Proportional Gain (Kc)"=w1932) -> (w1933:T9)
              n1460 = local write "Stroke PID Gains"(w1933) -> ()
            }
            frame 10 {
              n1461 = local write "Language Selection"(w1935) -> ()
            }
            frame 11 {
              n1462 = local write "CH-POWER +"(w1936) -> ()
            }
            frame 12 {
              n1463 = local write "CH-POWER -"(w1937) -> ()
            }
            frame 13 {
              n1464 = local write "CH-HEATER"(w1938) -> ()
            }
            frame 14 {
              n1465 = local write "CH-HUMIDITY WET"(w1939) -> ()
            }
            frame 15 {
              n1466 = local write "CH-HUMIDITY DRY"(w1940) -> ()
            }
            frame 16 {
              n1467 = local read "Stroke PID Gains"() -> (w1943:T9)
              n1468 = Bundle By Name(cluster=w1943, "Integral Time (Ti, min)"=w1941) -> (w1942:T9)
              n1469 = local write "Stroke PID Gains"(w1942) -> ()
            }
            frame 17 {
              n1470 = local write "AIR TEMP INTERCEPT:"(w1944) -> ()
            }
            frame 18 {
              n1471 = local write "TEMP INTERCEPT:"(w1945) -> ()
            }
            frame 19 {
              n1472 = local write "S.NO"(w1946) -> ()
            }
            frame 20 {
              n1473 = local write "Com Port 3"(w1947) -> ()
            }
            frame 21 {
              n1474 = local write "LvdtOff"(w1948) -> ()
            }
            frame 22 {
              n1475 = local write "C3 :"(w1949) -> ()
            }
            frame 23, Default {
            }
          }
        }
      }
    }
    n1476 = Select(t=u32 2500 ("milliseconds to wait"), s=w1896, f=u32 500 ("milliseconds to wait")) -> (s? t:f=w1894:u32)
    n1477 = Multiply(x=w1899, y=w1894) -> (x*y=w1901:dbl)
    n1478 = property on="FF Calibration g" class="WFGraph (strict)"("Visible"=w1890) -> ()  [unwired: 2 in, 2 out]
    n1479 = property on="Lift" class="Bool (strict)"("Visible"=w1890) -> ()  [unwired: 2 in, 2 out]
    n1480 = property on="Threshold" class="DigNum (strict)"("Visible"=w1890) -> ()  [unwired: 2 in, 2 out]
    n1481 = property on="Time slide" class="Slide (strict)"("Visible"=w1890) -> ()  [unwired: 2 in, 2 out]
    n1482 = call "Elapsed Time2"("Time Target (s)"=w1901, "Auto Reset"=TRUE) -> ("Time has Elapsed"=w1891:bool)  [unwired: 10 in, 7 out]
    n1483 = case shown="True" w1891 {
      frame False {
        # "79.77669138"
        # "2.3554"
        n1484 = local read "FRIC. FORCE :"() -> (w1954:dbl)
        n1485 = local read "FF cal val"() -> (w1951:dbl[])
        n1486 = Multiply(x=w1954, y=79.77669138) -> (x*y=w1953:dbl)
        n1487 = Multiply(x=w1951, y=w1953) -> (x*y=→"FF Calibration g":dbl[])
        "Err Count" <- 0 ("y")
      }
      frame True {
        n1488 = stacked-sequence {
          frame #0 {
            n1489 = stacked-sequence {
              frame #0 {
                "Lift" <- TRUE ("Lift")
              }
            }
          }
          frame #1 {
            w1966 = 2500 ("y")
            n1490 = local read "RUN"() -> (w1958:bool)
            n1491 = local read "FF1"() -> (w1961:dbl[])
            n1492 = case shown="False" w1958 {
              frame False {
                n1493 = local write "Frequency"(0.0 ("Frequency")) -> ()
              }
              frame True {
              }
            }
            n1494 = Array Size(array=w1961) -> (size(s)=w1960:i32)
            n1495 = local read "Ch1"() -> (w1957:dbl[])
            "Waveform Chart 2" <- w1957
            n1496 = call-poly <vilib>:"Mean.vi"("X"=w1957) -> ("mean"=→"Raw Mean":dbl)  [unwired: 1 out]
            n1497 = Insert Into Array(array=w1961, index=w1960, new element=w1957) -> (w1963:dbl[])
            n1498 = Array Size(array=w1963) -> (size(s)=w1967:i32)
            n1499 = Subtract(x=w1967, y=w1966) -> (x-y=w1965:i32)
            n1500 = Greater?(x=w1967, y=w1966) -> (0:w1968:bool)
            n1501 = case shown="True" w1968 {
              tunnel: w1965 -> [_ w1972]
              tunnel: [w1970 w1974] -> w1959
              tunnel: w1963 -> [w1970 w1973]
              frame False {
              }
              frame True {
                n1502 = Delete From Array(array=w1973, length=w1972, index=0) -> (array with subset deleted=w1974:dbl[])  [unwired: 1 out]
                "Numeric" <- w1972
              }
            }
            "FF1" <- w1959
            "PID Ref" <- TRUE ("PID Ref")
          }
          frame #2 {
          }
          frame #3 {
            # "CONVERT TO N"
            # "DATA PROCESSING"
            # "115 mV/N"
            n1503 = local read "RH Numeric:"() -> (w1980:dbl)
            n1504 = local read "HUMIDITY:"() -> (w1981:dbl)
            n1505 = local read "temp buf"() -> (w2042:dbl[])
            n1506 = local read "Air temp"() -> (w2040:dbl[])
            n1507 = local read "ecr buf"() -> (w2002:dbl[])
            n1508 = local read "Fric Val"() -> (w2045:dbl[])
            n1509 = case shown="True" "Reset Button" {
              frame False {
              }
              frame True {
                n1510 = local write "Reset Button"(FALSE) -> ()
                n1511 = local write "Captured Values"(dbl[][] [] ("Captured Values")) -> ()
                n1512 = local write "Best Fit"(dbl[] [] ("Best Fit")) -> ()
              }
            }
            n1513 = local read "TEMPERATURE :"() -> (w2023:dbl)
            n1514 = call-poly <vilib>:"Mean.vi"("X"=w2002) -> ("mean"=w1999:dbl)  [unwired: 1 out]
            n1515 = call-poly <vilib>:"Mean.vi"("X"=w2040) -> ("mean"=w2009:dbl)  [unwired: 1 out]
            "Raw air temp" <- w2009
            n1516 = call-poly <vilib>:"Mean.vi"("X"=w2042) -> ("mean"=w2011:dbl)  [unwired: 1 out]
            "Raw specimen temp" <- w2011
            n1517 = local read "TEMP INTERCEPT:"() -> (w2016:dbl)
            n1518 = Multiply(x=w1980, y=w1981) -> (x*y=→"Humidity ( %RH )" →"Hum" →"Hum 2":dbl)
            n1519 = Multiply(x=w2045, y=1.0) -> (x*y=w2046:dbl[])
            n1520 = local read "FRIC. FORCE :"() -> (w2039:dbl)
            n1521 = Multiply(x=w2011, y=w2023) -> (x*y=w2005:dbl)
            n1522 = local read "AIR TEMPERATURE :"() -> (w2024:dbl)
            n1523 = local read "RUN"() -> (w2036:bool)
            n1524 = Add(x=w2009, y="Offset Air Temp") -> (x+y=w2004:dbl)
            n1525 = local read "AIR TEMP INTERCEPT:"() -> (w2020:dbl)
            n1526 = case shown="\"0\", Default" "Calibrating" {
              tunnel: w2011 -> [w2065 _]
              tunnel: [w2065 w2066] -> w2010
              tunnel: w2009 -> [_ w2066]
              frame "0", Default {
              }
              frame "1" {
              }
            }
            n1527 = Multiply(x=w1999, y="ECR_Gain") -> (x*y=w1998:dbl)
            n1528 = Add(x=w2005, y=w2016) -> (x+y=w2021:dbl)
            n1529 = Multiply(x=w2039, y=79.77669138) -> (x*y=w2037:dbl)
            n1530 = Select(t=0.01 ("FF fil1"), s=w2036, f=0.1 ("FF fil1")) -> (s? t:f=w2032:dbl)
            n1531 = local read "ecr"() -> (w1993:dbl)
            n1532 = Multiply(x=w2004, y=w2024) -> (x*y=w2006:dbl)
            n1533 = Multiply(x=w2046, y=w2037) -> (x*y=w2043:dbl[])
            n1534 = Multiply(x=w1998, y=0.2) -> (x*y=w1991:dbl)
            n1535 = Multiply(x=0.8, y=w1993) -> (x*y=w1992:dbl)
            n1536 = call <vilib>:"Mean PtByPt.vi"("x"=w2021, "sample length"=10) -> ("mean"=w1982:dbl)  [unwired: 2 in, 1 out]
            "TEMP 2" <- w1982
            "TEMP 3" <- w1982
            n1537 = local read "AIR TEMP"() -> (w2029:dbl)
